vi "Write.vi"(8 "error in (no error)":errorcluster, 10 "Data":refnum<class "Data.lvclass">, 11 "Data Class in":refnum<class "Data Class.lvclass">) -> (0 "error out":errorcluster, 3 "Data Class out":refnum<class "Data Class.lvclass">)   [LabVIEW 2020, in "Data.lvlib" / "Data Class.lvclass"]
doc: "Write Data Class data."
uses:
  Data Class.lvclass
  Data.lvclass
  Cluster/Cluster.lvclass/Cluster.ctl
  Data Class.lvclass/Data Class.ctl
  Cluster/Cluster.lvclass
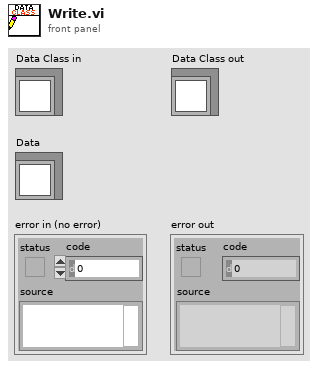
[diagram p1: front panel]
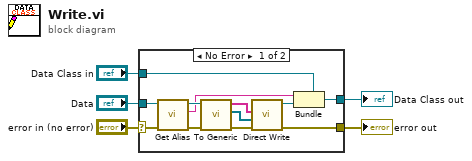
[diagram p0: block diagram]
diagram:
  n1 = case shown="No Error" "error in (no error)" {
    selector: "error in (no error)" -> [w11 w18]
    tunnel: [w8 w18] -> w4
    tunnel: [w12 w19] -> w2
    tunnel: "Data Class in" -> [w13 w19]
    tunnel: "Data" -> [w17 _]
    frame No Error {
      n2 = call-dynamic "Get Alias.vi"("error in (no error)"=w11, "Data in"=w17) -> ("error out"=w10:errorcluster, "Alias"=w7:string, "Data out"=w16:refnum<class "Data.lvclass">)  [unwired: 7 in]
      n3 = call-dynamic "To Generic.vi"("error in (no error)"=w10, "Data in"=w16) -> ("error out"=w9:errorcluster, "Generic Data"=w14:refnum<class "Generic Data.lvclass">[], "Data Name"=w15:string[])  [unwired: 7 in]
      n4 = call "Direct Write.vi"("error in (no error)"=w9, "Data Array"=w14, "Name Array"=w15) -> ("error out"=w8:errorcluster, "Cluster out"=w6:refnum<class "Cluster.lvclass">)  [unwired: 7 in]
      n5 = Bundle(cluster=w13, w7, w6) -> (w12:refnum<class "Data Class.lvclass">)
    }
    frame Error {
    }
  }
  "error out" <- w4
  "Data Class out" <- w2
